vi "DBL小数与整数（圆整）.vi"(11 "输入":dbl) -> (2 "小数部分":dbl, 3 "整数部分":dbl)   [LabVIEW 2012]
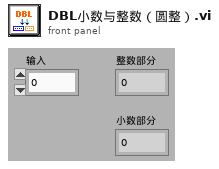
[diagram p1: front panel]
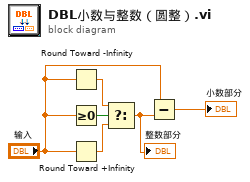
[diagram p0: block diagram]
diagram:
  n1 = Round Toward -Infinity(1:"输入") -> (0:w4:dbl)
  n2 = Greater Or Equal To 0?(x="输入") -> (x >= 0?=w6:bool)
  n3 = Round Toward +Infinity(x="输入") -> (ceil(x): smallest int >= x=w5:dbl)
  n4 = Select(t=w4, s=w6, f=w5) -> (s? t:f=w1:dbl)
  "整数部分" <- w1
  n5 = Subtract(x="输入", y=w1) -> (x-y=→"小数部分":dbl)
